vi "Utility Module 1.vi"(0 "Absolute start time (ms)":dbl=1500.0 format="%.3f", 1 "Static input":T4(array[cluster])=[{"Times"=[], "Voltages"=[], "Enable Ch"=TRUE, "Hinge Points"=0}, {"Times"=[], "Voltages"=[], "Enable Ch"=TRUE, "Hinge Points"=0}, {"Times"=[], "Voltages"=[], "Enable Ch"=TRUE, "Hinge Points"=0}, {"Times"=[], "Voltages"=[], "Enable Ch"=TRUE, "Hinge Points"=0}, {"Times"=[], "Voltages"=[], "Enable Ch"=TRUE, "Hinge Points"=0}, {"Times"=[], "Voltages"=[], "Enable Ch"=TRUE, "Hinge Points"=0}, {"Times"=[], "Voltages"=[], "Enable Ch"=TRUE, "Hinge Points"=0}, {"Times"=[], "Voltages"=[], "Enable Ch"=TRUE, "Hinge Points"=0}, {"Times"=[], "Voltages"=[], "Enable Ch"=TRUE, "Hinge Points"=0}, {"Times"=[], "Voltages"=[], "Enable Ch"=TRUE, "Hinge Points"=0}, {"Times"=[], "Voltages"=[], "Enable Ch"=TRUE, "Hinge Points"=0}, {"Times"=[], "Voltages"=[], "Enable Ch"=TRUE, "Hinge Points"=0}, {"Times"=[], "Voltages"=[], "Enable Ch"=TRUE, "Hinge Points"=0}, {"Times"=[], "Voltages"=[], "Enable Ch"=TRUE, "Hinge Points"=0}, {"Times"=[], "Voltages"=[], "Enable Ch"=TRUE, "Hinge Points"=0}, {"Times"=[], "Voltages"=[], "Enable Ch"=TRUE, "Hinge Points"=0}, {"Times"=[], "Voltages"=[], "Enable Ch"=TRUE, "Hinge Points"=0}, {"Times"=[], "Voltages"=[], "Enable Ch"=TRUE, "Hinge Points"=0}, {"Times"=[], "Voltages"=[], "Enable Ch"=TRUE, "Hinge Points"=0}, {"Times"=[], "Voltages"=[], "Enable Ch"=TRUE, "Hinge Points"=0}, {"Times"=[], "Voltages"=[], "Enable Ch"=TRUE, "Hinge Points"=0}, {"Times"=[], "Voltages"=[], "Enable Ch"=TRUE, "Hinge Points"=0}, {"Times"=[], "Voltages"=[], "Enable Ch"=TRUE, "Hinge Points"=0}, {"Times"=[], "Voltages"=[], "Enable Ch"=TRUE, "Hinge Points"=0}] {"Voltages" format="%.2f"; "Times" format="%.2f"}, 2 "Input":i64[][](array[numeric]), 3 "GPIB Input":T1(array[cluster]) {"Module" items=["TTL high                                                                                 ", "TTL low                          ", "Camera Strobe                   ", "CMOT", "Defaults                           ", "Fluorescence pulse           ", "IP trap                         ", "Kinetics OD image          ", "Kinetics picture", "Kinetics probe pulse", "MOT light only                ", "MOT off                                   ", "MOT on                         ", "Move cart                      ", "OD image                     ", "Optical pumping          ", "Picture                             ", "Probe Pulse", "Quadrupole trap             ", "IP off", "Utility Module 02           ", "Utility Module 03           ", "Molasses          ", "Utility Module 04     ", "Utility Module 05     ", "Utility Module 06     ", "Utility Module 07     ", "Utility Module 08     ", "Utility Module 09     ", "Utility Module 10     ", "Static DAC", "GPIB"]; "Abs Start Time" format="%.3f"}, 4 "Do this?":bool=TRUE) -> (5 "Static output":T4(array[cluster])=[{"Times"=[], "Voltages"=[], "Enable Ch"=TRUE, "Hinge Points"=0}, {"Times"=[], "Voltages"=[], "Enable Ch"=TRUE, "Hinge Points"=0}, {"Times"=[], "Voltages"=[], "Enable Ch"=TRUE, "Hinge Points"=0}, {"Times"=[], "Voltages"=[], "Enable Ch"=TRUE, "Hinge Points"=0}, {"Times"=[], "Voltages"=[], "Enable Ch"=TRUE, "Hinge Points"=0}, {"Times"=[], "Voltages"=[], "Enable Ch"=TRUE, "Hinge Points"=0}, {"Times"=[], "Voltages"=[], "Enable Ch"=TRUE, "Hinge Points"=0}, {"Times"=[], "Voltages"=[], "Enable Ch"=TRUE, "Hinge Points"=0}, {"Times"=[], "Voltages"=[], "Enable Ch"=TRUE, "Hinge Points"=0}, {"Times"=[], "Voltages"=[], "Enable Ch"=TRUE, "Hinge Points"=0}, {"Times"=[], "Voltages"=[], "Enable Ch"=TRUE, "Hinge Points"=0}, {"Times"=[], "Voltages"=[], "Enable Ch"=TRUE, "Hinge Points"=0}, {"Times"=[], "Voltages"=[], "Enable Ch"=TRUE, "Hinge Points"=0}, {"Times"=[], "Voltages"=[], "Enable Ch"=TRUE, "Hinge Points"=0}, {"Times"=[], "Voltages"=[], "Enable Ch"=TRUE, "Hinge Points"=0}, {"Times"=[], "Voltages"=[], "Enable Ch"=TRUE, "Hinge Points"=0}, {"Times"=[], "Voltages"=[], "Enable Ch"=TRUE, "Hinge Points"=0}, {"Times"=[], "Voltages"=[], "Enable Ch"=TRUE, "Hinge Points"=0}, {"Times"=[], "Voltages"=[], "Enable Ch"=TRUE, "Hinge Points"=0}, {"Times"=[], "Voltages"=[], "Enable Ch"=TRUE, "Hinge Points"=0}, {"Times"=[], "Voltages"=[], "Enable Ch"=TRUE, "Hinge Points"=0}, {"Times"=[], "Voltages"=[], "Enable Ch"=TRUE, "Hinge Points"=0}, {"Times"=[], "Voltages"=[], "Enable Ch"=TRUE, "Hinge Points"=0}, {"Times"=[1600.0, 1700.0], "Voltages"=[1.0, 2.0], "Enable Ch"=TRUE, "Hinge Points"=2}] {"Voltages" format="%.2f"; "Times" format="%.2f"}, 6 "Output":i64[][](array[numeric])=[[1700001, 3, 31, 0], [1700000, 3, 31, 1], [1600001, 3, 31, 0], [1600000, 3, 31, 1]], 7 "GPIB Output":T1(array[cluster]) {"Module" items=["TTL high                                                                                 ", "TTL low                          ", "Camera Strobe                   ", "CMOT", "Defaults                           ", "Fluorescence pulse           ", "IP trap                         ", "Kinetics OD image          ", "Kinetics picture", "Kinetics probe pulse", "MOT light only                ", "MOT off                                   ", "MOT on                         ", "Move cart                      ", "OD image                     ", "Optical pumping          ", "Picture                             ", "Probe Pulse", "Quadrupole trap             ", "IP off", "Utility Module 02           ", "Utility Module 03           ", "Molasses          ", "Utility Module 04     ", "Utility Module 05     ", "Utility Module 06     ", "Utility Module 07     ", "Utility Module 08     ", "Utility Module 09     ", "Utility Module 10     ", "Static DAC", "GPIB"]; "Abs Start Time" format="%.3f"})   [LabVIEW 2017]
uses:
  globals/Modules global.vi
panel:
  in  "Read/Write":bool
  in  "Do Write/Read":bool
  in  "Manual Array":T2(array[cluster])=[{"Time2 (ms)"="100", "Port2"=4, "Line2"=23, "Comments2"="", "Value2"=FALSE, "Enable2"=TRUE, "DAC value"="1"}, {"Time2 (ms)"="200", "Port2"=4, "Line2"=23, "Comments2"="", "Value2"=FALSE, "Enable2"=TRUE, "DAC value"="2"}] {"Line2" items=["0", "1", "2", "3", "4", "5", "6", "7", "8", "9", "10", "11", "12", "13", "14", "15", "16", "17", "18", "19", "20", "21", "22", "23", "24", "25", "26", "27", "28", "29", "30", "31"]; "Port2" items=["A", "B", "C", "D", "DAC", "GPIB"]}
  in  "filename":string="Utility Module 1"
  in  "Static DAC Linear Ramps":T3(array[cluster]) {"DAC Channel" items=["0", "1", "2", "3", "4", "5", "6", "7", "8", "9", "10", "11", "12", "13", "14", "15", "16", "17", "18", "19", "20", "21", "22", "23"]}
  # "Time                   Port        Line       Value  Enable  DAC voltage  Comments"
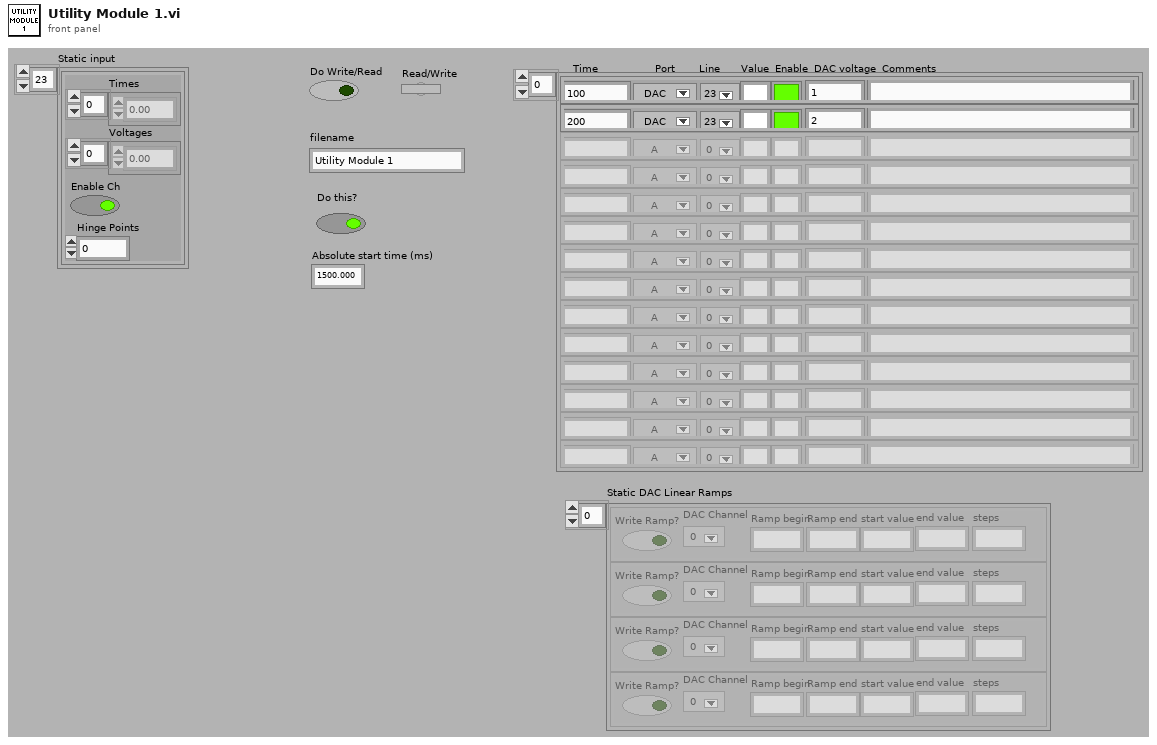
[diagram p1: front panel]
types:
  T1 = cluster{"Enable":bool, "Abs Start Time":dbl, "Module":u16, "String":string, "Array":string[]}[]
  T2 = cluster{"Time2 (ms)":string, "Port2":u16, "Line2":u16, "Comments2":string, "Value2":bool, "Enable2":bool, "DAC value":string}[]
  T3 = cluster{"Write Ramp?":bool, "DAC Channel":i16, "Ramp begin":string, "Ramp end":string, "start value":string, "end value":string, "steps":string}[]
  T4 = cluster{"Times":dbl[], "Voltages":dbl[], "Enable Ch":bool, "Hinge Points":u8}[]
  T5 = cluster{"Manual Array":cluster{"Time2 (ms)":dbl, "Port2":u16, "Line2":u16, "Comments2":string, "Value2":bool, "Enable2":bool, "DAC value":dbl}[], "Static DAC Linear Ramps":cluster{"Write Ramp?":bool, "DAC Channel":i16, "Ramp begin":dbl, "Ramp end":dbl, "start value":dbl, "end value":dbl, "steps":i16}[]}
  T6 = cluster{"Time2 (ms)":dbl, "Port2":u16, "Line2":u16, "Comments2":string, "Value2":bool, "Enable2":bool, "DAC value":dbl}[]
  T7 = cluster{"Write Ramp?":bool, "DAC Channel":i16, "Ramp begin":dbl, "Ramp end":dbl, "start value":dbl, "end value":dbl, "steps":i16}[]
  T8 = cluster{"Time2 (ms)":string, "Port2":u16, "Line2":u16, "Comments2":string, "Value2":bool, "Enable2":bool, "DAC value":string}
  T9 = cluster{"Write Ramp?":bool, "DAC Channel":i16, "Ramp begin":string, "Ramp end":string, "start value":string, "end value":string, "steps":string}
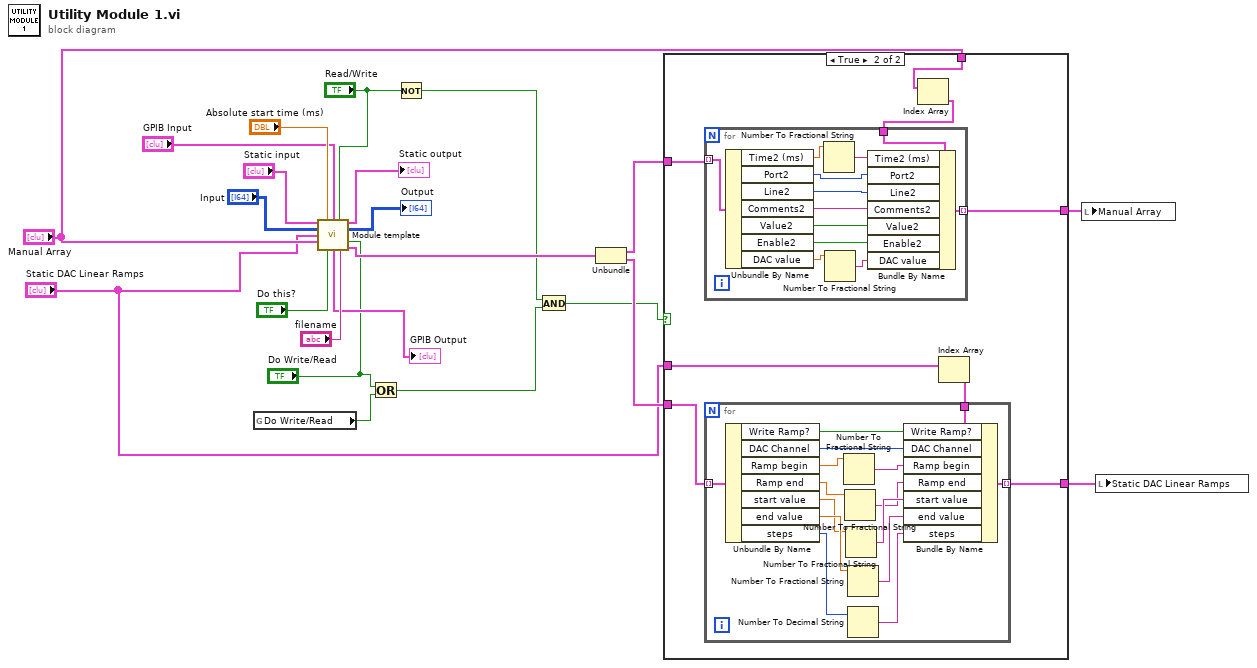
[diagram p0: block diagram]
diagram:
  n1 = global read "Modules global.vi" "Do Write/Read"() -> (w8:bool)
  n2 = call "Module template.vi"("Static input"="Static input", "Absolute start time (ms)"="Absolute start time (ms)", "GPIB Input"="GPIB Input", "Read/Write"="Read/Write", "Input"="Input", "Static DAC Linear Ramps"="Static DAC Linear Ramps", "Manual Array"="Manual Array", "Do Write/Read"="Do Write/Read", "Do this?"="Do this?", "filename"="filename") -> ("Static output"=→"Static output":T4, "Output"=→"Output":i64[][], "GPIB Output"=→"GPIB Output":T1, "Saved Cluster"=w16:T5)  [unwired: 2 in]
  n3 = Or(x="Do Write/Read", y=w8) -> (x .or. y?=w5:bool)
  n4 = Not(x="Read/Write") -> (.not. x?=w6:bool)
  n5 = And(x=w6, y=w5) -> (x .and. y?=w4:bool)
  n6 = Unbundle(w16) -> ("Manual Array"=w11:T6, "Static DAC Linear Ramps"=w10:T7)
  n7 = case shown="True" w4 {
    tunnel: w11 -> [_ w32]
    tunnel: w10 -> [_ w31]
    tunnel: "Manual Array" -> [w23 w30]
    tunnel: "Static DAC Linear Ramps" -> [w24 w28]
    tunnel: [w23 w26] -> w2
    tunnel: [w24 w25] -> w1
    frame False {
    }
    frame True {
      n8 = Index Array(array=w30) -> (element=w29:T8)  [unwired: 1 in]
      n9 = for {
        tunnel: w32 -> [w59] mode=indexing
        tunnel: w29 -> [w58]
        tunnel: [w48] -> w26 mode=indexing
        n10 = Unbundle By Name(w59) -> ("Time2 (ms)"=w51:dbl, "Port2"=w56:u16, "Line2"=w55:u16, "Comments2"=w54:string, "Value2"=w53:bool, "Enable2"=w52:bool, "DAC value"=w50:dbl)
        n11 = Number To Fractional String(number=w51) -> (F-format string=w57:string)  [unwired: 3 in]
        n12 = Number To Fractional String(number=w50) -> (F-format string=w49:string)  [unwired: 3 in]
        n13 = Bundle By Name(cluster=w58, "Time2 (ms)"=w57, "Port2"=w56, "Line2"=w55, "Comments2"=w54, "Value2"=w53, "Enable2"=w52, "DAC value"=w49) -> (w48:T8)
      }
      n14 = Index Array(array=w28) -> (element=w27:T9)  [unwired: 1 in]
      n15 = for {
        tunnel: w31 -> [w47] mode=indexing
        tunnel: w27 -> [w46]
        tunnel: [w33] -> w25 mode=indexing
        n16 = Unbundle By Name(w47) -> ("Write Ramp?"=w45:bool, "DAC Channel"=w44:i16, "Ramp begin"=w34:dbl, "Ramp end"=w37:dbl, "start value"=w39:dbl, "end value"=w41:dbl, "steps"=w43:i16)
        n17 = Number To Fractional String(number=w34) -> (F-format string=w35:string)  [unwired: 3 in]
        n18 = Number To Fractional String(number=w37) -> (F-format string=w36:string)  [unwired: 3 in]
        n19 = Number To Fractional String(number=w39) -> (F-format string=w38:string)  [unwired: 3 in]
        n20 = Number To Fractional String(number=w41) -> (F-format string=w40:string)  [unwired: 3 in]
        n21 = Number To Decimal String(number=w43) -> (decimal integer string=w42:string)  [unwired: 1 in]
        n22 = Bundle By Name(cluster=w46, "Write Ramp?"=w45, "DAC Channel"=w44, "Ramp begin"=w35, "Ramp end"=w36, "start value"=w38, "end value"=w40, "steps"=w42) -> (w33:T9)
      }
    }
  }
  n23 = local write "Manual Array"(w2) -> ()
  n24 = local write "Static DAC Linear Ramps"(w1) -> ()
